vi "send.vi"(5 "sender":refnum<class "identifying queue.lvclass">, 7 "enqueue command":T1, 8 "error in":errorcluster, 9 "timeout in ms (-1)":i32=-1, 10 "message":refnum<class "communicator message.lvclass">, 11 "message connection in":refnum<class "identifying queue.lvclass">) -> (0 "error out":errorcluster, 1 "timed out?":bool)   [LabVIEW 2015, in "identifying queue.lvclass"]
uses:
  identifying queue.lvclass
  message/communicator message.lvclass
  enqueue variety.ctl
  identifying queue.lvclass/identifying queue.ctl
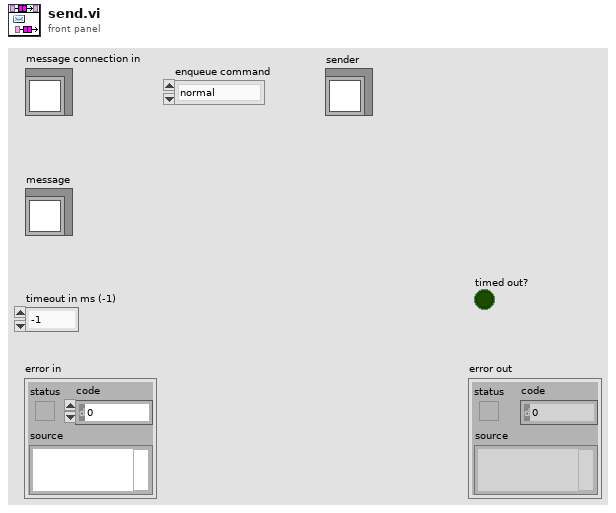
[diagram p1: front panel]
types:
  T1 = typedef "identifying queue.lvclass/enqueue variety.ctl" = enum16{"normal", "lossy", "priority"}
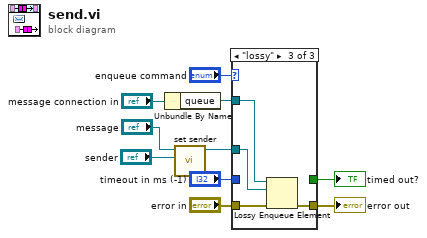
[diagram p0: block diagram]
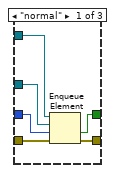
[diagram p2: hidden frame]
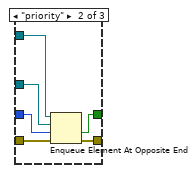
[diagram p3: hidden frame]
diagram:
  n1 = Unbundle By Name("message connection in") -> ("queue"=w8:refnum<queue>)
  n2 = call "set sender.vi"("sender"="sender", "message in"="message") -> ("message out"=w3:refnum<class "communicator message.lvclass">)  [unwired: 9 in]
  n3 = case shown="\"lossy\"" "enqueue command" {
    tunnel: w8 -> [w16 w22 w26]
    tunnel: "error in" -> [w15 w21 w23]
    tunnel: [w12 w18 w25] -> w6
    tunnel: "timeout in ms (-1)" -> [w14 w20 _]
    tunnel: w3 -> [w13 w19 w24]
    tunnel: [w11 w17 _] -> w1
    frame "normal" {
      n4 = Enqueue Element(queue=w16, element=w13, timeout in ms (-1)=w14, error in (no error)=w15) -> (timed out?=w11:bool, error out=w12:errorcluster)  [unwired: 1 out]
    }
    frame "priority" {
      n5 = Enqueue Element At Opposite End(queue=w22, element=w19, timeout in ms (-1)=w20, error in (no error)=w21) -> (timed out?=w17:bool, error out=w18:errorcluster)  [unwired: 1 out]
    }
    frame "lossy" {
      n6 = Lossy Enqueue Element(queue=w26, element=w24, error in (no error)=w23) -> (error out=w25:errorcluster)  [unwired: 3 out]
    }
  }
  "error out" <- w6
  "timed out?" <- w1
